vi "Plotter.vi"() -> ()   [LabVIEW 2019]
uses:
  <vilib>/Instr/_visa.llb/VISA Flush IO Buffer Mask.ctl
  <vilib>/Instr/_visa.llb/VISA Configure Serial Port (Instr).vi
  <vilib>/measure/NI_MABase.lvlib
  <vilib>/ptbypt/NI_PtbyPt.lvlib
panel:
  out "TX Period, ms":u32
  out "Boolean 7":bool
  out "CO2 Flow":dbl(graph) caption="ADC CH2 Давление на выходе аппарата"
  out "Boolean 6":bool
  in  "Duty cycle,\n       %":sgl(slide)=50.0 scale=0.0..100.0
  in  "UART TX Period":dbl(slide)=5.0 scale=5.0..1000.0
  out "OK":bool
  in  "COM port":refnum<visa-resource-name>
  in  "CO2 ON":bool
  out "Boolean 3":bool
  in  "Air ON":bool
  in  "AUTO":bool=TRUE
  in  "CO2 Flow":u16(slide)=2000 scale=0.0..4095.0 scale format="%4d"
  out "TX, Bytes":i32
  out "Write buffer":string
  in  "Air Flow":u16(slide)=2000 scale=0.0..4095.0
  in  "Breathing rate,\n       1/min":dbl(slide)=60.0 step=0.1 scale=2.0..150.0
  out "Ток пропорциональных клапанов":cluster{dbl, dbl}(graph)
  out "Air Flow":dbl(graph) caption="ADC CH2 Давление на выходе аппарата"
  out "Read buffer":string
  out "RX, Bytes":i32
  in  "stop":bool
  # "OFF"
  # "AUTO"
  # "AUTO"
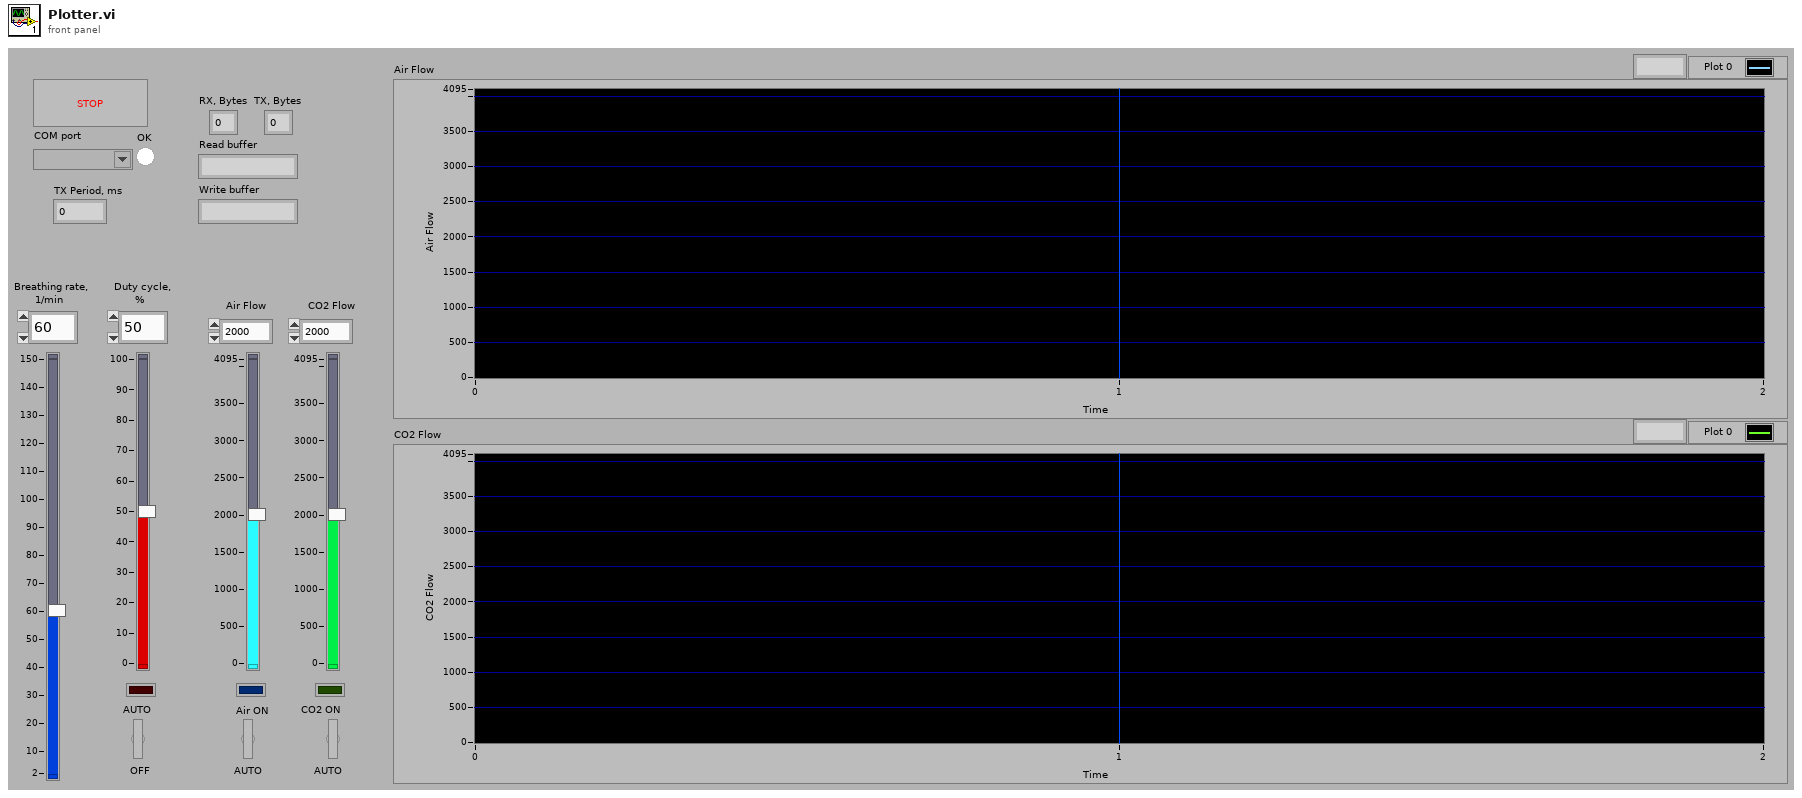
[diagram p1: front panel]
types:
  T1 = typedef "VISA Flush IO Buffer Mask.ctl" = u16
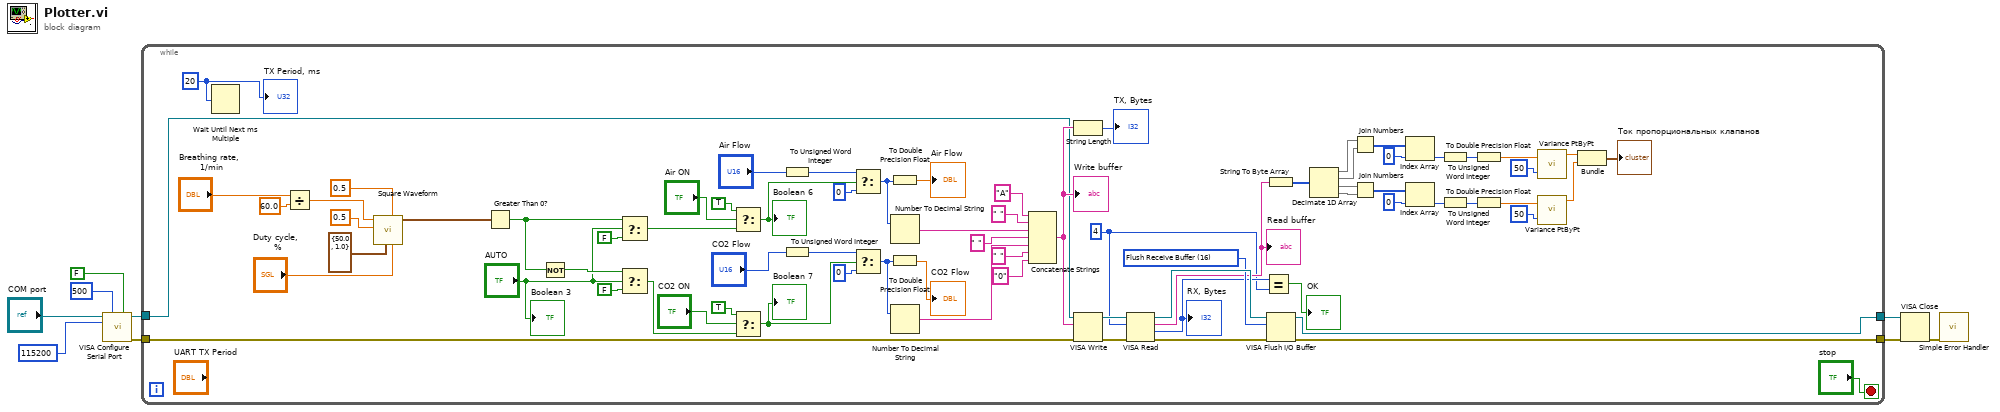
[diagram p0: block diagram]
diagram:
  n1 = call-poly "VISA Configure Serial Port"("VISA resource name"="COM port", "timeout (10sec)"=u32 500, "Enable Termination\nChar (T)"=FALSE ("Enable Termination\nChar (T)"), "baud rate (9600)"=u32 115200 ("baud rate (115200)")) -> ("VISA resource name out"=w6:refnum<visa-resource-name>, "error out"=w5:errorcluster)  [unwired: 10 in]
  n2 = while {
    tunnel: w6 -> [w39]
    tunnel: w5 -> [w83]
    tunnel: [w77] -> w3
    tunnel: [w79] -> w2
    stop <- "stop" stop-if-true
    w21 = u32 20 ("millisecond multiple")
    w76 = T1 16 items=["Flush Receive Buffer"=16, "Write Transmit Buffer to Device"=32, "Flush Receive Buffer (No I/O)"=64, "Flush Transmit Buffer"=128] ("Mask")
    w54 = u32 4 ("byte count")
    n3 = Wait Until Next ms Multiple(millisecond multiple=w21) -> ()  [unwired: 1 out]
    n4 = Divide(x="Breathing rate,\n       1/min", y=60.0) -> (x/y=w12:dbl)
    n5 = call <vilib>:"Square Waveform.vi"("duty cycle (%)"="Duty cycle,\n       %", "offset"=0.5, "sampling info"=cluster{"Fs":dbl, "#s":dbl} {"Fs"=50.0, "#s"=1.0}, "amplitude"=0.5, "frequency"=w12) -> ("signal out"=w23:waveform(dbl))  [unwired: 5 in, 1 out]
    n6 = Greater Than 0?(x=w23) -> (x > 0?=w24:bool)
    n7 = Not(x=w24) -> (.not. x?=w35:bool)
    n8 = Select(t=w24, s="AUTO", f=FALSE) -> (s? t:f=w32:bool)
    n9 = Select(t=w35, s="AUTO", f=FALSE) -> (s? t:f=w28:bool)
    n10 = Select(t=TRUE, s="Air ON", f=w32) -> (s? t:f=w31:bool)
    "Boolean 6" <- w31
    n11 = Select(t=TRUE, s="CO2 ON", f=w28) -> (s? t:f=w27:bool)
    "Boolean 7" <- w27
    n12 = To Unsigned Word Integer(number="Air Flow") -> (unsigned 16bit integer=w66:u16)
    n13 = To Unsigned Word Integer(number="CO2 Flow") -> (unsigned 16bit integer=w42:u16)
    n14 = Select(t=w66, s=w31, f=u16 0) -> (s? t:f=w44:u16)
    n15 = Select(t=w42, s=w27, f=u16 0) -> (s? t:f=w41:u16)
    n16 = To Double Precision Float(number=w44) -> (double precision float=→"Air Flow":dbl)
    n17 = Number To Decimal String(number=w44) -> (decimal integer string=w49:string)  [unwired: 1 in]
    n18 = To Double Precision Float(number=w41) -> (double precision float=→"CO2 Flow":dbl)
    n19 = Number To Decimal String(number=w41) -> (decimal integer string=w46:string)  [unwired: 1 in]
    n20 = Concatenate Strings("A" ("write buffer"), " " ("write buffer"), w49, " " ("write buffer"), w46, " " ("string"), "0" ("string")) -> (w63:string)
    "Write buffer" <- w63
    n21 = String Length(string=w63) -> (length=→"TX, Bytes":i32)
    n22 = VISA Write(VISA resource name=w39, write buffer=w63, error in (no error)=w83) -> (VISA resource name out=w81:refnum<visa-resource-name>, error out=w82:errorcluster)  [unwired: 1 out]
    n23 = VISA Read(VISA resource name=w81, byte count=w54, error in (no error)=w82) -> (VISA resource name out=w80:refnum<visa-resource-name>, read buffer=w75:string, return count=w55:u32, error out=w78:errorcluster)
    "RX, Bytes" <- w55
    "Read buffer" <- w75
    n24 = Equal?(x=w55, y=w54) -> (x = y?=→"OK":bool)
    n25 = String To Byte Array(string=w75) -> (unsigned byte array=w74:u8[])
    n26 = VISA Flush I/O Buffer(VISA resource name=w80, mask (16)=w76, error in (no error)=w78) -> (VISA resource name out=w79:refnum<visa-resource-name>, error out=w77:errorcluster)
    n27 = Decimate 1D Array(w74) -> (w58:u8[], w59:u8[], w57:u8[], w56:u8[])
    n28 = Join Numbers(hi=w58, lo=w59) -> ((hi.lo)=w68:u16[])
    n29 = Join Numbers(hi=w57, lo=w56) -> ((hi.lo)=w71:u16[])
    n30 = Index Array(array=w68, index=0) -> (element=w70:u16)
    n31 = Index Array(array=w71, index=0) -> (element=w43:u16)
    n32 = To Unsigned Word Integer(number=w70) -> (unsigned 16bit integer=w52:u16)
    n33 = To Unsigned Word Integer(number=w43) -> (unsigned 16bit integer=w69:u16)
    n34 = To Double Precision Float(number=w52) -> (double precision float=w17:dbl)
    n35 = To Double Precision Float(number=w69) -> (double precision float=w14:dbl)
    n36 = call <vilib>:"Variance PtByPt.vi"("x"=w17, "sample length"=50) -> ("mean"=w16:dbl)  [unwired: 1 in, 2 out]
    n37 = call <vilib>:"Variance PtByPt.vi"("x"=w14, "sample length"=50) -> ("mean"=w13:dbl)  [unwired: 1 in, 2 out]
    n38 = Bundle("mean"=w16, "mean"=w13) -> (→"Ток пропорциональных клапанов":cluster{"mean":dbl, "mean":dbl})  [unwired: 1 in]
    "Boolean 3" <- "AUTO"
    "TX Period, ms" <- w21
  }
  n39 = VISA Close(VISA resource name=w2, error in (no error)=w3) -> (error out=w4:errorcluster)
  n40 = call <vilib>:"Simple Error Handler.vi"("error in (no error)"=w4) -> ()  [unwired: 1 in, 8 out]
